vi "Test VI Source Separated.vi"(8 "error in (no error)":errorcluster, 10 "VI Refnum":refnum<vi>, 11 "testStateMachineUtilities in":refnum<class "testStateMachineUtilities.lvclass">) -> (0 "error out":errorcluster, 3 "testStateMachineUtilities out":refnum<class "testStateMachineUtilities.lvclass">)   [LabVIEW 2020]
uses:
  testStateMachineUtilities/testStateMachineUtilities.lvclass
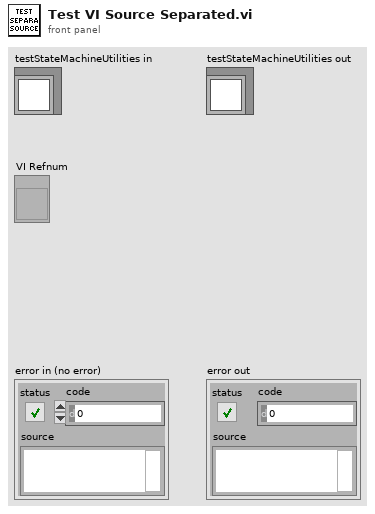
[diagram p1: front panel]
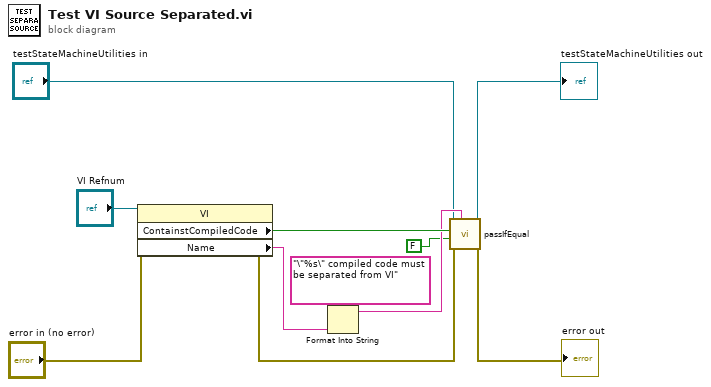
[diagram p0: block diagram]
diagram:
  n1 = property class="VI"(reference="VI Refnum", error in="error in (no error)") -> (error out=w9:errorcluster, "ContainstCompiledCode"=w11:bool, "Name"=w10:string)  [unwired: 1 out]
  n2 = Format Into String(format string="\"%s\" compiled code must be separated from VI", w10) -> (resulting string=w6:string)  [unwired: 2 in, 1 out]
  n3 = call-dynamic "passIfEqual.vi"("custom report message (\"\")"=w6, "error in (no error)"=w9, "y"=FALSE, "x"=w11, "TestCase in"="testStateMachineUtilities in") -> ("error out"=→"error out":errorcluster, "TestCase out"=→"testStateMachineUtilities out":refnum<class "testStateMachineUtilities.lvclass">)  [unwired: 5 in]
